vi "GV_ZoomHorizontalPerform.vi"(8 "error in (no error)":errorcluster, 9 "Coords":T1, 11 "Gviewer in":refnum<class "Gviewer.lvclass">) -> (0 "error out":errorcluster, 3 "Gviewer out":refnum<class "Gviewer.lvclass">)   [LabVIEW 2020, in "Sgraph_lib_V1.lvlib" / "Gviewer.lvclass"]
doc: "Andre Koelewijn, 8 may 2021\n\nPerform the horizontal zoom action when the mouse button is released"
uses:
  Gviewer.lvclass
  <vilib>/Utility/miscctls.llb/LVPoint32TypeDef.ctl
  Gviewer.lvclass/Gviewer.ctl
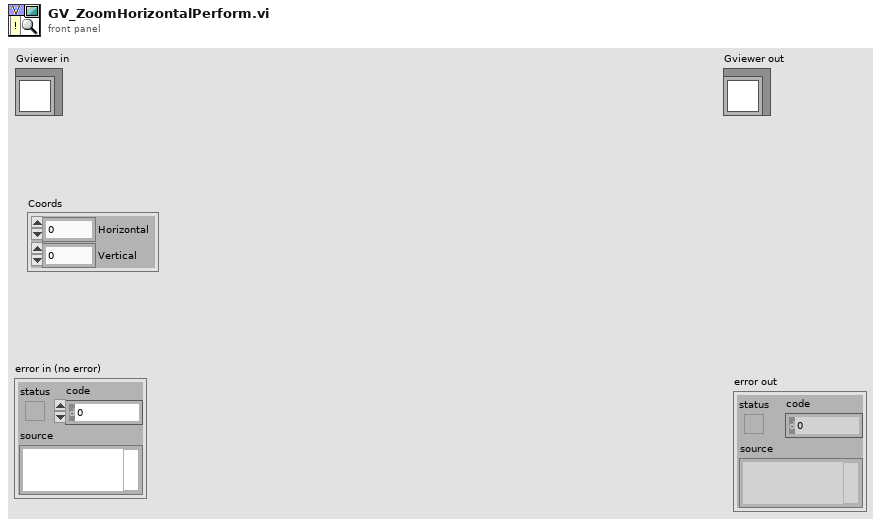
[diagram p1: front panel]
types:
  T1 = typedef "LVPoint32TypeDef.ctl" = cluster{"Horizontal":i32, "Vertical":i32}
  T2 = cluster{"left":i16, "top":i16, "right":i16, "bottom":i16}
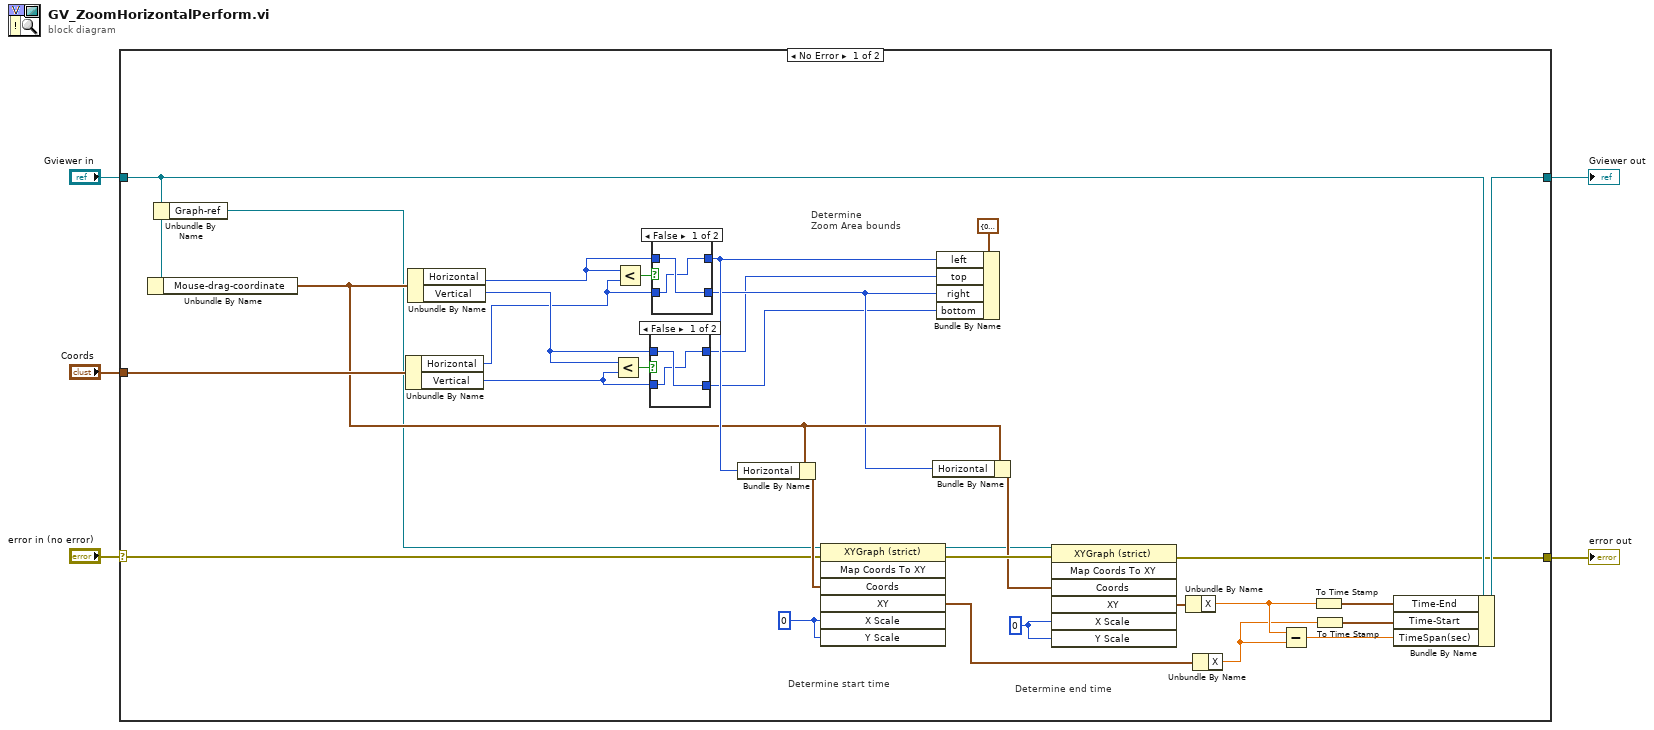
[diagram p0: block diagram]
diagram:
  n1 = case shown="No Error" "error in (no error)" {
    selector: "error in (no error)" -> [w6 w46]
    tunnel: [w8 w46] -> w4
    tunnel: [w9 w45] -> w2
    tunnel: "Gviewer in" -> [w18 w45]
    tunnel: "Coords" -> [w21 _]
    frame No Error {
      w29 = 0 ("X Scale")
      w28 = 0 ("X Scale")
      # "Determine\nZoom Area bounds"
      # "Determine start time"
      # "Determine end time"
      n2 = Unbundle By Name(w18) -> ("Mouse-drag-coordinate"=w20:T1)
      n3 = Unbundle By Name(w18) -> ("Graph-ref"=w7:refnum<vi>)
      n4 = Unbundle By Name(w21) -> ("Horizontal"=w11:i32, "Vertical"=w10:i32)
      n5 = Unbundle By Name(w20) -> ("Horizontal"=w13:i32, "Vertical"=w12:i32)
      n6 = Less?(x=w12, y=w10) -> (x < y?=w31:bool)
      n7 = Less?(x=w13, y=w11) -> (x < y?=w30:bool)
      n8 = case shown="False" w31 {
        tunnel: w12 -> [w38 w40]
        tunnel: [w37 w40] -> w14
        tunnel: [w38 w39] -> w15
        tunnel: w10 -> [w37 w39]
        frame False {
        }
        frame True {
        }
      }
      n9 = case shown="False" w30 {
        tunnel: w13 -> [w42 w44]
        tunnel: [w41 w44] -> w36
        tunnel: [w42 w43] -> w19
        tunnel: w11 -> [w41 w43]
        frame False {
        }
        frame True {
        }
      }
      n10 = Bundle By Name(cluster=w20, "Horizontal"=w36) -> (w32:T1)
      n11 = invoke class="XYGraph (strict)" method="Map Coords To XY"(reference=w7, error in=w6, "Coords"=w32, "X Scale"=w28, "Y Scale"=w28) -> (reference out=w33:refnum<vi>, error out=w35:errorcluster, "XY"=w16:cluster{"X":dbl, "Y":dbl})  [unwired: 2 in, 4 out]
      n12 = Bundle By Name(cluster=w20, "Horizontal"=w19) -> (w34:T1)
      n13 = Bundle By Name(cluster=T2 {"left"=0, "top"=0, "right"=0, "bottom"=0} ("rect"), "left"=w36, "top"=w14, "right"=w19, "bottom"=w15) -> ()  [unwired: 1 out]
      n14 = invoke class="XYGraph (strict)" method="Map Coords To XY"(reference=w33, error in=w35, "Coords"=w34, "X Scale"=w29, "Y Scale"=w29) -> (error out=w8:errorcluster, "XY"=w17:cluster{"X":dbl, "Y":dbl})  [unwired: 2 in, 5 out]
      n15 = Unbundle By Name(w17) -> ("X"=w25:dbl)
      n16 = Unbundle By Name(w16) -> ("X"=w24:dbl)
      n17 = Subtract(x=w25, y=w24) -> (x-y=w26:dbl)
      n18 = To Time Stamp(1:w25) -> (0:w22:timestamp)
      n19 = To Time Stamp(1:w24) -> (0:w23:timestamp)
      n20 = Bundle By Name(cluster=w18, "Time-End"=w22, "Time-Start"=w23, "TimeSpan(sec)"=w26) -> (w9:refnum<class "Gviewer.lvclass">)
    }
    frame Error {
    }
  }
  "error out" <- w4
  "Gviewer out" <- w2
